vi "VeristandStart.vi"(1 "error in (no error)":errorcluster, 2 "Open VeriStand Timeout (s)":i32=120, 3 "Gateway IP Address (\"\": localhost)":string) -> (0 "error out":errorcluster)   [LabVIEW 2020, in "ni-veristand-steps-runtime-lib.lvlib"]
uses:
  ni-veristand-steps-runtime-lib.lvlib
  controls/VeriStand dotNet References.ctl
  <vilib>/NI VeriStand/Execution/ModelManager/ModelManagerAPI.ctl
  <vilib>/NI VeriStand/Execution/AlarmManager/AlarmManagerAPI.ctl
  <vilib>/NI VeriStand/Execution/ChannelFaultManager/ChannelFaultAPI.ctl
  <vilib>/NI VeriStand/Execution/Workspace/WorkspaceAPI.ctl
  <vilib>/NI VeriStand/Execution/Project/Project Ref.ctl
  <vilib>/Utility/error.llb/Error Cluster From Error Code.vi
  <vilib>/ErrorRing/Error Ring.xnode
  <vilib>/NI VeriStand/Execution/Workspace/NI_VS Workspace ExecutionAPI.lvlib
  NationalInstruments.VeriStand.ClientAPI
  <vilib>/NI VeriStand/Execution/Project/NI_VS Project ExecutionAPI.lvlib
  <vilib>/NI VeriStand/Execution/ChannelFaultManager/NI_VS ChannelFault ExecutionAPI.lvlib
  <vilib>/NI VeriStand/Execution/AlarmManager/NI_VS AlarmManager ExecutionAPI.lvlib
  <vilib>/NI VeriStand/Execution/ModelManager/NI_VS ModelManager ExecutionAPI.lvlib
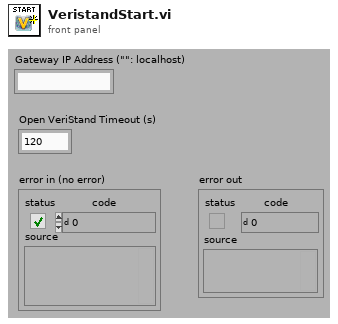
[diagram p1: front panel]
types:
  T1 = typedef "ni-veristand-steps-runtime-lib.lvlib/VeriStand dotNet References.ctl" = cluster{"ModelManager":T2, "AlarmManager":T3, "ChannelFault":T4, "WorkspaceManager":T5, "Project Ref":T6}
  T2 = typedef "NI_VS ModelManager ExecutionAPI.lvlib/ModelManagerAPI.ctl" = refnum<k24>
  T3 = typedef "NI_VS AlarmManager ExecutionAPI.lvlib/AlarmManagerAPI.ctl" = refnum<k24>
  T4 = typedef "NI_VS ChannelFault ExecutionAPI.lvlib/ChannelFaultAPI.ctl" = refnum<k24>
  T5 = typedef "NI_VS Workspace ExecutionAPI.lvlib/WorkspaceAPI.ctl" = refnum<k24>
  T6 = typedef "NI_VS Project ExecutionAPI.lvlib/Project Ref.ctl" = refnum<k24>
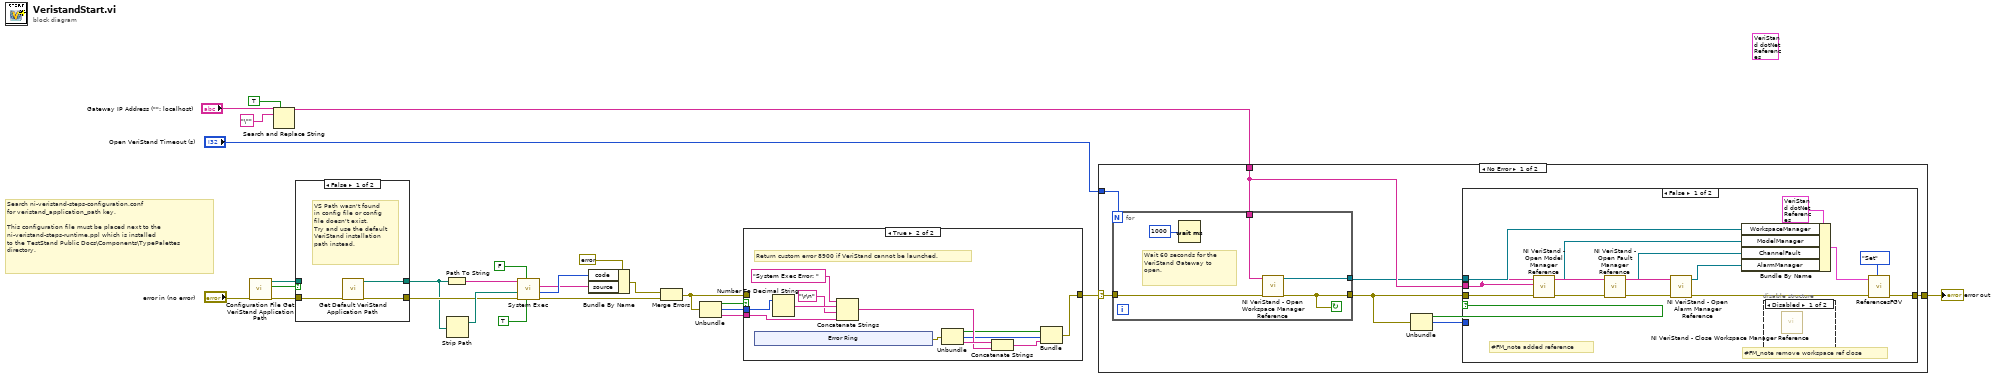
[diagram p0: block diagram]
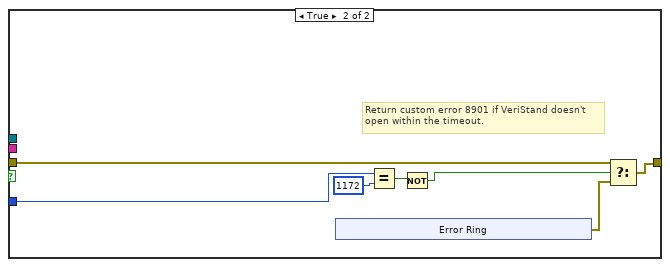
[diagram p3: hidden frame]
diagram:
  (unwired) T1 {"ModelManager"=refnum, "AlarmManager"=refnum, "ChannelFault"=refnum, "WorkspaceManager"=refnum, "Project Ref"=refnum} ("VeriStand dotNET Refs")
  # "Search ni-veristand-steps-configuration.conf \nfor veristand_application_path key.\n\nThis configuration file must be placed next to the\nni-veristand-steps-runtime.ppl which is installed\nto the TestStand Public Docs\\Components\\TypePalettes\ndirectory."
  n1 = call "Configuration File Get VeriStand Application Path.vi"("error in (no error)"="error in (no error)") -> ("error out"=w16:errorcluster, "Found?"=w14:bool, "VeriStand Application Path"=w15:path)  [unwired: 8 in]
  n2 = Search and Replace String(replace all?=TRUE ("replace all? (F)"), input string="Gateway IP Address (\"\": localhost)", search string="\"") -> (result string=w1:string)  [unwired: 5 in, 3 out]
  n3 = case shown="False" w14 {
    tunnel: w16 -> [w29 w30]
    tunnel: w15 -> [_ w31]
    tunnel: [w27 w31] -> w11
    tunnel: [w28 w30] -> w12
    frame False {
      # "VS Path wasn't found\nin config file or config\nfile doesn't exist.\nTry and use the default\nVeriStand installation\npath instead."
      n4 = call "Get Default VeriStand Application Path.vi"("error in (no error)"=w29) -> ("error out"=w28:errorcluster, "Default VeriStand App Path"=w27:path)  [unwired: 9 in]
    }
    frame True {
    }
  }
  n5 = Path To String(path=w11) -> (string=w10:string)
  n6 = Strip Path(path=w11) -> (stripped path=w13:path)  [unwired: 1 out]
  n7 = call <vilib>:"System Exec.vi"("run minimized? (F)"=TRUE, "wait until completion? (T)"=FALSE, "error in (no error)"=w12, "working directory"=w13, "command line"=w10) -> ("error out"=w21:errorcluster, "return code"=w23:i32, "standard error"=w18:string)  [unwired: 3 in, 1 out]
  n8 = Bundle By Name(cluster=errorcluster {"status"=FALSE, "code"=0, "source"=""} ("error in (no error)"), "code"=w23, "source"=w18) -> (w22:errorcluster)
  n9 = Merge Errors(w22, w21) -> (w6:errorcluster)
  n10 = Unbundle(w6) -> ("status"=w9:bool, "code"=w8:i32, "source"=w7:string)
  n11 = case shown="True" w9 {
    tunnel: [w32 w33] -> w5
    tunnel: w8 -> [_ w43]
    tunnel: w7 -> [_ w39]
    tunnel: w6 -> [w32 _]
    frame False {
    }
    frame True {
      # "Return custom error 8900 if VeriStand cannot be launched."
      n12 = xnode "Error Ring"() -> ("error out"=w44:errorcluster)
      n13 = Number To Decimal String(number=w43) -> (decimal integer string=w41:string)  [unwired: 1 in]
      n14 = Concatenate Strings("System Exec Error: " ("string"), w41, "\r\n", w39) -> (w37:string)
      n15 = Unbundle(w44) -> ("status"=w36:bool, "code"=w35:i32, "source"=w38:string)
      n16 = Concatenate Strings(w38, w37) -> (w34:string)
      n17 = Bundle("status"=w36, "code"=w35, w34) -> (w33:cluster{"status":bool, "code":i32, string})  [unwired: 1 in]
    }
  }
  n18 = case shown="No Error" w5 {
    selector: w5 -> [w53 w88]
    tunnel: [w55 w88] -> w20
    tunnel: "Open VeriStand Timeout (s)" -> [w54 _]
    tunnel: w1 -> [w51 _]
    frame No Error {
      n19 = for {
        N: w54 -> [_]
        tunnel: [w85] -> w50
        tunnel: [w86] -> w52
        tunnel: w53 -> [w84]
        tunnel: w51 -> [w83]
        stop <- w86 continue-if-true
        # "Wait 60 seconds for the VeriStand Gateway to open."
        n20 = Wait (ms)(milliseconds to wait=u32 1000) -> ()  [unwired: 1 out]
        n21 = call <vilib>:"NI VeriStand - Open Workspace Manager Reference.vi"("error in (no error)"=w84, "Gateway IP Address (\"\": localhost)"=w83) -> ("error out"=w86:errorcluster, "WorkspaceManager"=w85:T5)  [unwired: 8 in]
      }
      n22 = Unbundle(w52) -> ("status"=w57:bool, "code"=w56:i32)  [unwired: 1 out]
      n23 = case shown="False" w57 {
        tunnel: w56 -> [_ w77]
        tunnel: w52 -> [w66 w74]
        tunnel: [w59 w75] -> w55
        tunnel: w51 -> [w65 _]
        tunnel: w50 -> [w70 _]
        frame False {
          # "#FM_note remove workspace ref close"
          # "#FM_note added reference"
          n24 = call <vilib>:"NI VeriStand - Open Model Manager Reference.vi"("error in (no error)"=w66, "Gateway IP Address (\"\": localhost)"=w65) -> ("error out"=w67:errorcluster, "ModelManager"=w62:T2)  [unwired: 8 in]
          n25 = call <vilib>:"NI VeriStand - Open Fault Manager Reference.vi"("error in (no error)"=w67, "Gateway IP Address (\"\": localhost)"=w65) -> ("error out"=w68:errorcluster, "ChannelFault"=w63:T4)  [unwired: 8 in]
          n26 = call <vilib>:"NI VeriStand - Open Alarm Manager Reference.vi"("error in (no error)"=w68, "Gateway IP Address (\"\": localhost)"=w65) -> ("error out"=w60:errorcluster, "AlarmManager"=w64:T3)  [unwired: 8 in]
          n27 = Bundle By Name(cluster=T1 {"ModelManager"=refnum, "AlarmManager"=refnum, "ChannelFault"=refnum, "WorkspaceManager"=refnum, "Project Ref"=refnum} ("input cluster"), "WorkspaceManager"=w70, "ModelManager"=w62, "ChannelFault"=w63, "AlarmManager"=w64) -> (w58:T1)
          n28 = disable-structure shown="Disabled" {
            frame Disabled {
              n29 = call <vilib>:"NI VeriStand - Close Workspace Manager Reference.vi"() -> ()  [unwired: 11 in, 1 out]
            }
            frame Enabled {
            }
          }
          n30 = call "ReferencesFGV.vi"("Get/Set"=enum16{"Get", "Set"}."Set", "error in (no error)"=w60, "VeriStand dotNET Refs"=w58) -> ("error out"=w59:errorcluster)  [unwired: 7 in, 1 out]
        }
        frame True {
          # "Return custom error 8901 if VeriStand doesn't\nopen within the timeout."
          n31 = xnode "Error Ring"() -> ("error out"=w71:errorcluster)
          n32 = Equal?(x=w77, y=1172) -> (x = y?=w73:bool)
          n33 = Not(x=w73) -> (.not. x?=w72:bool)
          n34 = Select(t=w74, s=w72, f=w71) -> (s? t:f=w75:errorcluster)
        }
      }
    }
    frame Error {
    }
  }
  "error out" <- w20
